vi "Scripting_RemoveDynamicDispatchInGoop2VIs.vi"(0 "ViRef":refnum<vi>, 1 "ForceDynamicDispatch":bool, 5 "error in (no error)":errorcluster) -> (15 "DynamicDispatch":bool, 19 "error out":errorcluster)   [LabVIEW 2020]
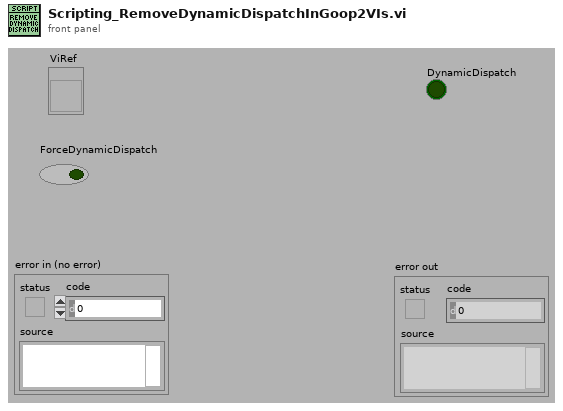
[diagram p1: front panel]
types:
  T1 = cluster{"FindDMRef":refnum<vi>, "Case":refnum<vi>, "DynamicDispatch":bool, "FindVi":path, "RegVi":path}
  T2 = enum16{"Invalid Wire Rule", "Required", "Recommended", "Optional", "Dynamic Dispatch"}
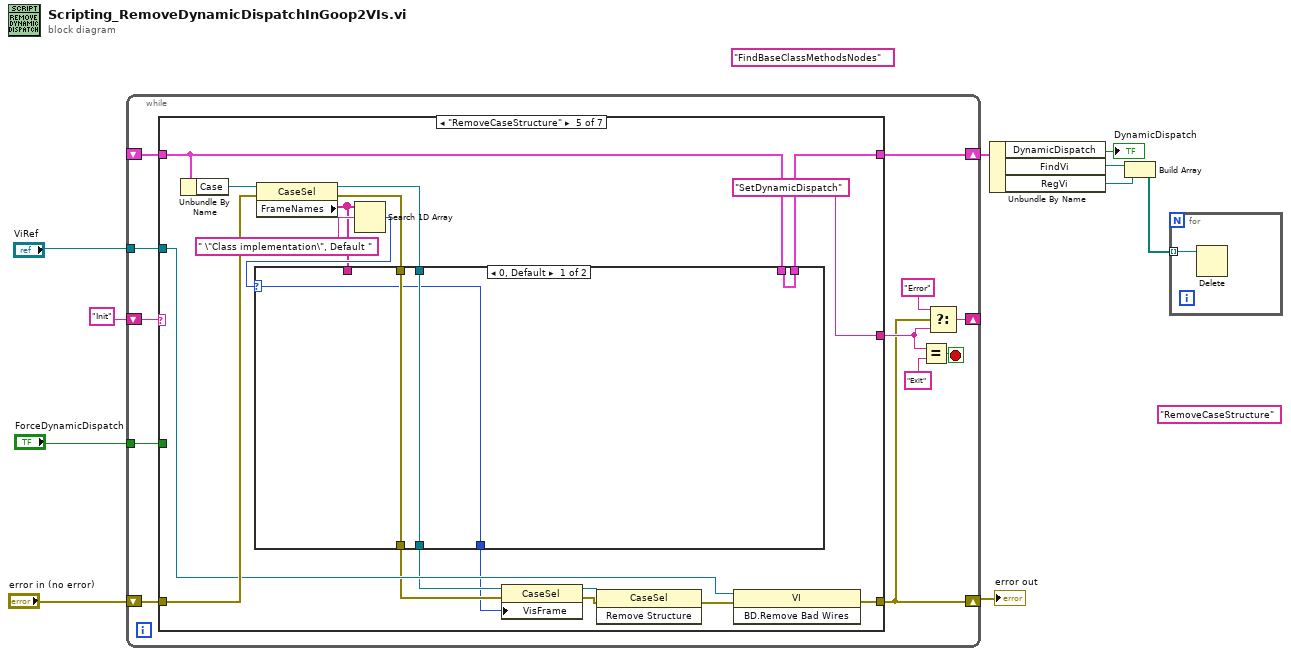
[diagram p0: block diagram]
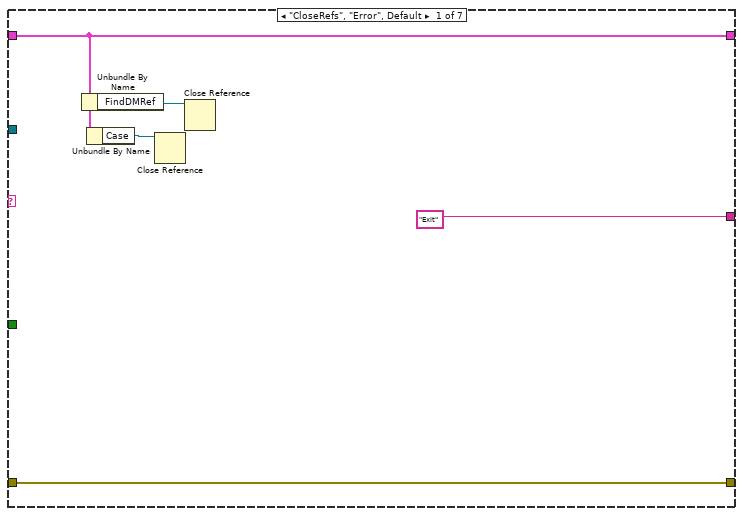
[diagram p2: hidden frame]
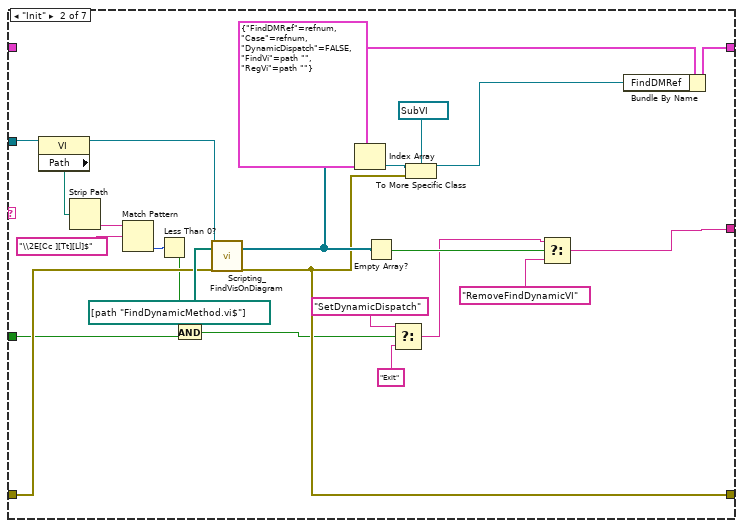
[diagram p3: hidden frame]
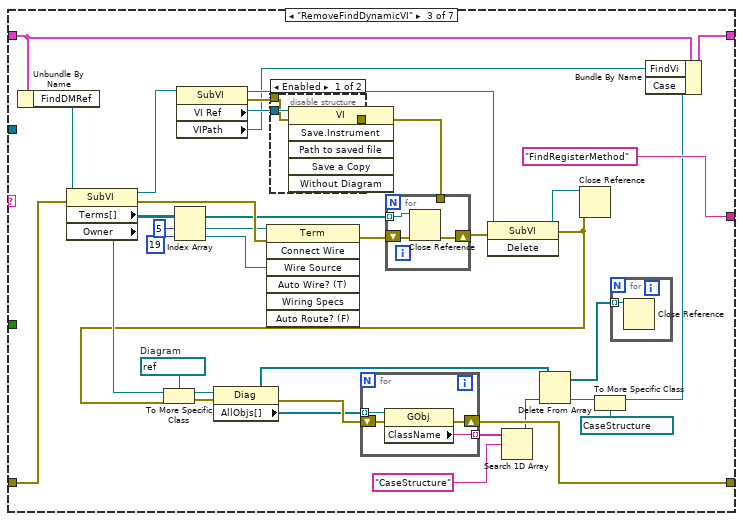
[diagram p4: hidden frame]
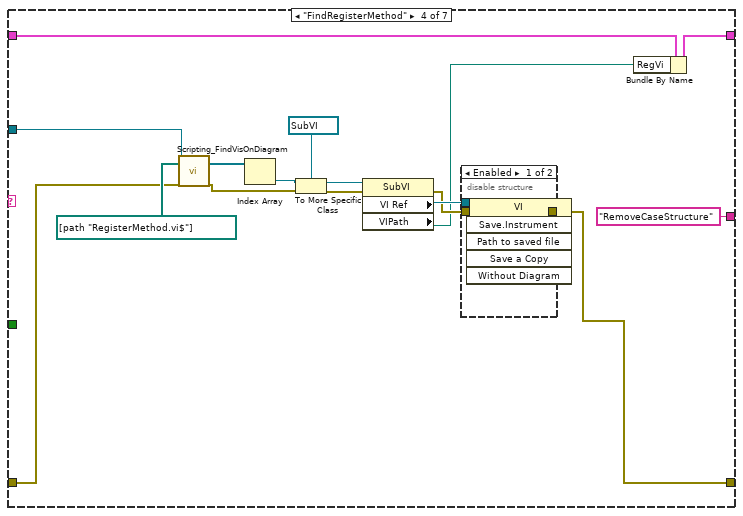
[diagram p6: hidden frame]
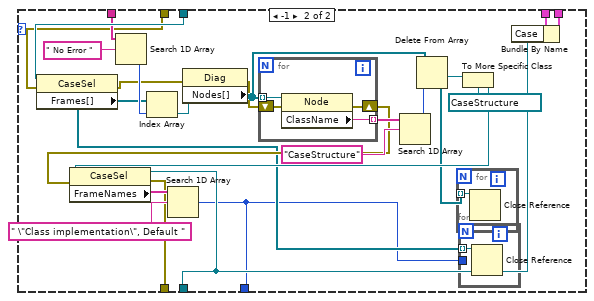
[diagram p8: hidden frame]
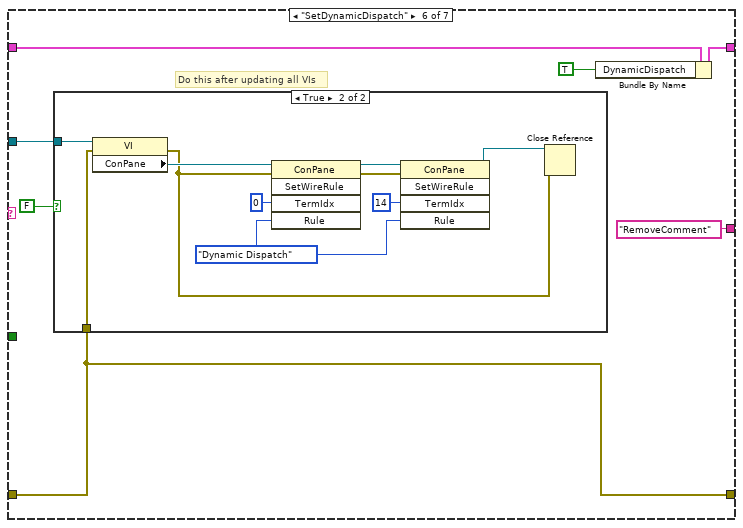
[diagram p9: hidden frame]
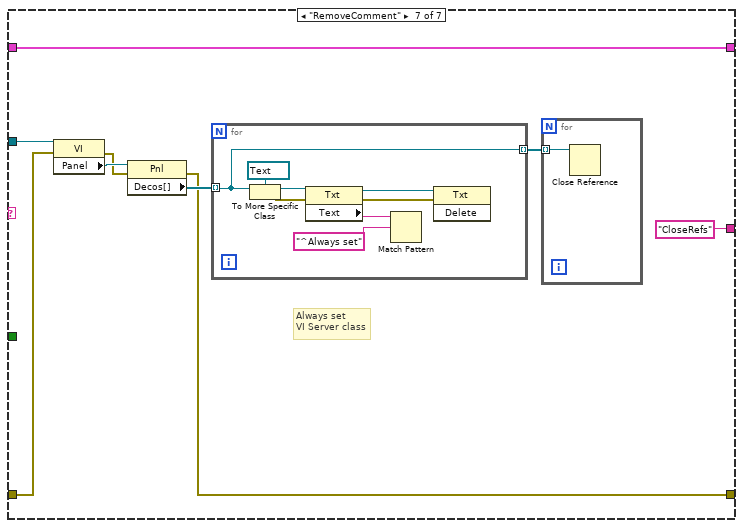
[diagram p11: hidden frame]
diagram:
  (unwired) "FindBaseClassMethodsNodes"
  (unwired) "RemoveCaseStructure"
  n1 = while {
    shift-right: [w15] -> w8
    shift-left: "error in (no error)" -> [w22]
    shift-right: [w20] -> _
    shift-left: "Init" -> [w21]
    shift-right: [w14] -> w5
    shift-left: _ -> [w13]
    tunnel: "ViRef" -> [w12]
    tunnel: "ForceDynamicDispatch" -> [w11]
    stop <- w19 stop-if-true
    n2 = case shown="\"RemoveCaseStructure\"" w21 {
      tunnel: w22 -> [w27 w40 w78 w112 w131 w176 w192]
      tunnel: [w27 w43 w66 w102 w129 w176 w190] -> w15
      tunnel: ["Exit" w46 "FindRegisterMethod" "RemoveCaseStructure" "SetDynamicDispatch" "RemoveComment" "CloseRefs"] -> w16
      tunnel: [w25 w50 w86 w100 w119 w173 w189] -> w14
      tunnel: w13 -> [w25 _ w84 w101 w120 w174 w189]
      tunnel: w12 -> [_ w34 _ w113 w128 w177 w196]
      tunnel: w11 -> [_ w36 _ _ _ _ _]
      frame "CloseRefs", "Error", Default {
        n3 = Unbundle By Name(w25) -> ("FindDMRef"=w24:refnum<vi>)
        n4 = Unbundle By Name(w25) -> ("Case"=w23:refnum<vi>)
        n5 = Close Reference(reference=w23) -> ()  [unwired: 1 in, 1 out]
        n6 = Close Reference(reference=w24) -> ()  [unwired: 1 in, 1 out]
      }
      frame "Init" {
        n7 = property class="VI"(reference=w34) -> (reference out=w35:refnum<vi>, "Path"=w33:path)  [unwired: 1 in, 1 out]
        n8 = Strip Path(path=w33) -> (name=w32:string)  [unwired: 1 out]
        n9 = Match Pattern(string=w32, regular expression="\\2E[Cc ][Tt][Ll]$") -> (offset past match=w29:i32)  [unwired: 1 in, 3 out]
        n10 = Less Than 0?(x=w29) -> (x < 0?=w28:bool)
        n11 = And(x=w28, y=w36) -> (x .and. y?=w30:bool)
        n12 = call "Scripting_FindVisOnDiagram.vi"("ViRef"=w35, "VIsToSerachFor/ViName"=path[] [path "FindDynamicMethod.vi$"] ("TypeDefControlsToSerachFor"), "error in (no error)"=w40) -> ("VisFound"=w45:refnum<vi>[], "error out"=w43:errorcluster)  [unwired: 15 in]
        n13 = Index Array(array=w45) -> (element=w44:refnum<vi>)  [unwired: 1 in]
        n14 = Empty Array?(array=w45) -> (empty?=w48:bool)
        n15 = Select(t="SetDynamicDispatch", s=w30, f="Exit") -> (s? t:f=w39:string)
        n16 = To More Specific Class(target class=refnum<vi> refnum ("element"), reference=w44, error in=w43) -> (specific class reference=w41:refnum<vi>)  [unwired: 1 out]
        n17 = Select(t=w39, s=w48, f="RemoveFindDynamicVI") -> (s? t:f=w46:string)
        n18 = Bundle By Name(cluster=T1 {"FindDMRef"=refnum, "Case"=refnum, "DynamicDispatch"=FALSE, "FindVi"=path "", "RegVi"=path ""}, "FindDMRef"=w41) -> (w50:T1)
      }
      frame "RemoveFindDynamicVI" {
        w72 = refnum<vi> refnum  # Diagram
        n19 = Unbundle By Name(w84) -> ("FindDMRef"=w77:refnum<vi>)
        n20 = property class="SubVI"(reference=w77, error in=w78) -> (reference out=w58:refnum<vi>, error out=w83:errorcluster, "Terms[]"=w75:refnum<vi>[], "Owner"=w60:refnum<vi>)
        n21 = Index Array(array=w75, index #1=5 ("index"), index #2=19 ("index")) -> (element #1=w79:refnum<vi>, element #2=w82:refnum<vi>)
        n22 = property class="SubVI"(reference=w58) -> (reference out=w54:refnum<vi>, error out=w56:errorcluster, "VI Ref"=w57:refnum<vi>, "VIPath"=w52:path)  [unwired: 1 in]
        n23 = invoke class="Term" method="Connect Wire"(reference=w79, error in=w83, "Wire Source"=w82) -> (error out=w76:errorcluster)  [unwired: 4 in, 6 out]
        n24 = disable-structure shown="Enabled" {
          disable-tunnel: w57 -> [w89 _]
          disable-tunnel: w56 -> [w88 w90]
          disable-tunnel: [w87 w90] -> w55
          frame Enabled {
            n25 = invoke class="VI" method="Save.Instrument"(reference=w89, error in=w88) -> (error out=w87:errorcluster)  [unwired: 4 in, 5 out]
          }
          frame Disabled {
          }
        }
        n26 = for {
          shift-right: [w96] -> w74
          shift-left: w76 -> [w98]
          tunnel: w75 -> [w97] mode=indexing
          tunnel: w55 -> [_]
          n27 = Close Reference(reference=w97, error in (no error)=w98) -> (error out=w96:errorcluster)
        }
        n28 = invoke class="SubVI" method="Delete"(reference=w54, error in=w74) -> (reference out=w73:refnum<vi>, error out=w53:errorcluster)  [unwired: 1 in, 1 out]
        n29 = To More Specific Class(target class=w72, reference=w60, error in=w53) -> (specific class reference=w70:refnum<vi>, error out=w71:errorcluster)
        n30 = property class="Diag"(reference=w70, error in=w71) -> (error out=w67:errorcluster, "AllObjs[]"=w64:refnum<vi>[])  [unwired: 1 out]
        n31 = for {
          tunnel: w64 -> [w95] mode=indexing
          tunnel: [w94] -> w69 mode=indexing
          shift-right: [w92] -> w66
          shift-left: w67 -> [w93]
          n32 = property class="GObj"(reference=w95, error in=w93) -> (error out=w92:errorcluster, "ClassName"=w94:string)  [unwired: 1 out]
        }
        n33 = Search 1D Array(1D array=w69, element="CaseStructure") -> (index of element=w65:i32)  [unwired: 1 in]
        n34 = Delete From Array(array=w64, index=w65) -> (deleted portion=w63:refnum<vi>, array with subset deleted=w59:refnum<vi>[])  [unwired: 1 in]
        n35 = Close Reference(reference=w73, error in (no error)=w53) -> ()  [unwired: 1 out]
        n36 = To More Specific Class(target class=refnum<vi> refnum ("Case"), reference=w63) -> (specific class reference=w61:refnum<vi>)  [unwired: 1 in, 1 out]
        n37 = for {
          tunnel: w59 -> [w91] mode=indexing
          n38 = Close Reference(reference=w91) -> ()  [unwired: 1 in, 1 out]
        }
        n39 = Bundle By Name(cluster=w84, "FindVi"=w52, "Case"=w61) -> (w86:T1)
      }
      frame "FindRegisterMethod" {
        n40 = call "Scripting_FindVisOnDiagram.vi"("ViRef"=w113, "VIsToSerachFor/ViName"=path[] [path "RegisterMethod.vi$"] ("TypeDefControlsToSerachFor"), "error in (no error)"=w112) -> ("VisFound"=w109:refnum<vi>[], "error out"=w104:errorcluster)  [unwired: 15 in]
        n41 = Index Array(array=w109) -> (element=w111:refnum<vi>)  [unwired: 1 in]
        n42 = To More Specific Class(target class=refnum<vi> refnum ("element"), reference=w111, error in=w104) -> (specific class reference=w106:refnum<vi>, error out=w105:errorcluster)
        n43 = property class="SubVI"(reference=w106, error in=w105) -> (error out=w107:errorcluster, "VI Ref"=w108:refnum<vi>, "VIPath"=w99:path)  [unwired: 1 out]
        n44 = disable-structure shown="Enabled" {
          disable-tunnel: w108 -> [w117 _]
          disable-tunnel: w107 -> [w116 w118]
          disable-tunnel: [w115 w118] -> w102
          frame Enabled {
            n45 = invoke class="VI" method="Save.Instrument"(reference=w117, error in=w116) -> (error out=w115:errorcluster)  [unwired: 4 in, 5 out]
          }
          frame Disabled {
          }
        }
        n46 = Bundle By Name(cluster=w101, "RegVi"=w99) -> (w100:T1)
      }
      frame "RemoveCaseStructure" {
        n47 = Unbundle By Name(w120) -> ("Case"=w135:refnum<vi>)
        n48 = property class="CaseSel"(reference=w135, error in=w131) -> (reference out=w126:refnum<vi>, error out=w122:errorcluster, "FrameNames"=w123:string[])
        n49 = Search 1D Array(1D array=w123, element=" \"Class implementation\", Default ") -> (index of element=w127:i32)  [unwired: 1 in]
        n50 = case shown="0, Default" w127 {
          selector: w127 -> [w138 _]
          tunnel: w122 -> [w140 w152]
          tunnel: [w140 w148] -> w124
          tunnel: w126 -> [w139 w165]
          tunnel: [w139 w144] -> w125
          tunnel: w123 -> [_ w164]
          tunnel: [w138 w141] -> w121
          tunnel: w120 -> [w137 w162]
          tunnel: [w137 w161] -> w119
          frame 0, Default {
          }
          frame -1 {
            n51 = property class="CaseSel"(reference=w165, error in=w152) -> (error out=w153:errorcluster, "Frames[]"=w142:refnum<vi>[])  [unwired: 1 out]
            n52 = Search 1D Array(1D array=w164, element=" No Error ") -> (index of element=w160:i32)  [unwired: 1 in]
            n53 = Index Array(array=w142, index=w160) -> (element=w156:refnum<vi>)
            n54 = property class="Diag"(reference=w156, error in=w153) -> (error out=w154:errorcluster, "Nodes[]"=w155:refnum<vi>[])  [unwired: 1 out]
            n55 = for {
              tunnel: w155 -> [w171] mode=indexing
              tunnel: [w170] -> w157 mode=indexing
              shift-right: [w168] -> w149
              shift-left: w154 -> [w169]
              n56 = property class="Node"(reference=w171, error in=w169) -> (error out=w168:errorcluster, "ClassName"=w170:string)  [unwired: 1 out]
            }
            n57 = Search 1D Array(1D array=w157, element="CaseStructure") -> (index of element=w159:i32)  [unwired: 1 in]
            n58 = Delete From Array(array=w155, index=w159) -> (deleted portion=w146:refnum<vi>, array with subset deleted=w143:refnum<vi>[])  [unwired: 1 in]
            n59 = for {
              tunnel: w143 -> [w167] mode=indexing
              n60 = Close Reference(reference=w167) -> ()  [unwired: 1 in, 1 out]
            }
            n61 = To More Specific Class(target class=refnum<vi> refnum ("Case"), reference=w146) -> (specific class reference=w145:refnum<vi>)  [unwired: 1 in, 1 out]
            n62 = property class="CaseSel"(reference=w145, error in=w149) -> (reference out=w144:refnum<vi>, error out=w148:errorcluster, "FrameNames"=w151:string[])
            n63 = Search 1D Array(1D array=w151, element=" \"Class implementation\", Default ") -> (index of element=w141:i32)  [unwired: 1 in]
            n64 = for {
              tunnel: w142 -> [w166] mode=indexing
              tunnel: w141 -> [_]
              n65 = Close Reference(reference=w166) -> ()  [unwired: 1 in, 1 out]
            }
            n66 = Bundle By Name(cluster=w162, "Case"=w144) -> (w161:T1)
          }
        }
        n67 = property class="CaseSel"(reference=w125, error in=w124, "VisFrame"=w121) -> (reference out=w133:refnum<vi>, error out=w132:errorcluster)
        n68 = invoke class="CaseSel" method="Remove Structure"(reference=w133, error in=w132) -> (error out=w130:errorcluster)  [unwired: 1 in, 2 out]
        n69 = invoke class="VI" method="BD.Remove Bad Wires"(reference=w128, error in=w130) -> (error out=w129:errorcluster)  [unwired: 1 in, 2 out]
      }
      frame "SetDynamicDispatch" {
        # "Do this after updating all VIs"
        n70 = case shown="True" FALSE {
          tunnel: w177 -> [_ w182]
          tunnel: w176 -> [_ w179]
          frame False {
          }
          frame True {
            w183 = T2."Dynamic Dispatch" ("Rule")
            n71 = property class="VI"(reference=w182, error in=w179) -> (error out=w180:errorcluster, "ConPane"=w184:refnum<vi>)  [unwired: 1 out]
            n72 = invoke class="ConPane" method="SetWireRule"(reference=w184, error in=w180, "TermIdx"=u32 0 ("Terminal Index"), "Rule"=w183) -> (reference out=w188:refnum<vi>, error out=w187:errorcluster)  [unwired: 1 in, 3 out]
            n73 = invoke class="ConPane" method="SetWireRule"(reference=w188, error in=w187, "TermIdx"=u32 14 ("Terminal Index"), "Rule"=w183) -> (reference out=w181:refnum<vi>)  [unwired: 1 in, 4 out]
            n74 = Close Reference(reference=w181, error in (no error)=w180) -> ()  [unwired: 1 out]
          }
        }
        n75 = Bundle By Name(cluster=w174, "DynamicDispatch"=TRUE) -> (w173:T1)
      }
      frame "RemoveComment" {
        # "Always set\nVI Server class"
        n76 = property class="VI"(reference=w196, error in=w192) -> (error out=w191:errorcluster, "Panel"=w195:refnum<vi>)  [unwired: 1 out]
        n77 = property class="Pnl"(reference=w195, error in=w191) -> (error out=w190:errorcluster, "Decos[]"=w194:refnum<vi>[])  [unwired: 1 out]
        n78 = for {
          tunnel: w194 -> [w199] mode=indexing
          tunnel: [w199] -> w193 mode=indexing
          n79 = To More Specific Class(target class=refnum<vi> refnum ("reference"), reference=w199) -> (specific class reference=w205:refnum<vi>, error out=w200:errorcluster)  [unwired: 1 in]
          n80 = property class="Txt"(reference=w205, error in=w200) -> (reference out=w202:refnum<vi>, error out=w201:errorcluster, "Text"=w204:string)
          n81 = Match Pattern(string=w204, regular expression="^Always set") -> ()  [unwired: 1 in, 4 out]
          n82 = invoke class="Txt" method="Delete"(reference=w202, error in=w201) -> ()  [unwired: 1 in, 3 out]
        }
        n83 = for {
          tunnel: w193 -> [w198] mode=indexing
          n84 = Close Reference(reference=w198) -> ()  [unwired: 1 in, 1 out]
        }
      }
    }
    n85 = Equal?(x=w16, y="Exit") -> (x = y?=w19:bool)
    n86 = Select(t="Error", s=w15, f=w16) -> (s? t:f=w20:string)
  }
  "error out" <- w8
  n87 = Unbundle By Name(w5) -> ("DynamicDispatch"=→"DynamicDispatch":bool, "FindVi"=w3:path, "RegVi"=w2:path)
  n88 = Build Array(w3, w2) -> (w1:path[])
  n89 = for {
    tunnel: w1 -> [w207] mode=indexing
    n90 = Delete(path (use dialog)=w207) -> ()  [unwired: 4 in, 3 out]
  }
